vi "GFITS_WriteAmps.vi"(0 "fd":u64, 1 "filemsg":string, 2 "multimple extensions":bool, 3 "amplifiers":u64, 4 "eleRead":u32, 5 "error in":errorcluster, 6 "expID":string, 7 "Database RefNum in":T1, 8 "nodeID":string, 9 "headers":bool=TRUE, 10 "logfile":path, 11 "number of keywords":i32[](array[numeric])) -> (14 "file reference out":u64, 15 "return value":i32, 16 "after expID":string, 17 "image name out":string, 19 "error out":errorcluster)   [LabVIEW 2016]
uses:
  DBSHAND/private/vis/DatabaseHand_RefNum.ctl
  Common/public/vis/CMN_FVAR_action.ctl
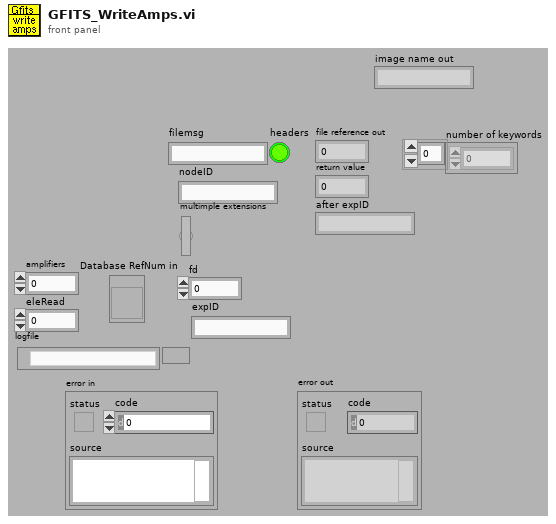
[diagram p1: front panel]
types:
  T1 = typedef "DatabaseHand_RefNum.ctl" = refnum<vi>
  T2 = typedef "CMN_FVAR_action.ctl" = enum16{"read", "write"}
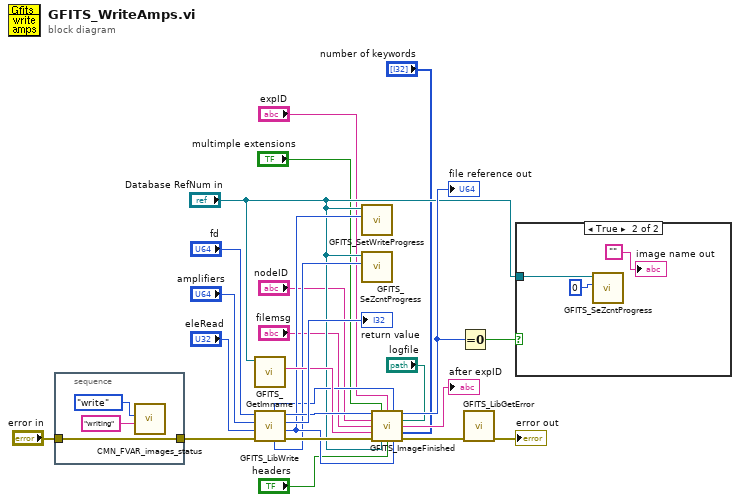
[diagram p0: block diagram]
diagram:
  n1 = stacked-sequence {
    tunnel: "error in" -> [w26]
    tunnel: [w26] -> w13
    frame #0 {
      n2 = call "CMN_FVAR_images_status.vi"("value in"="writing", "action"=CMN_FVAR_action."write") -> ()  [unwired: 9 out]
    }
  }
  n3 = call "GFITS_GetImname.vi"("Database RefNum"="Database RefNum in") -> ("name"=w21:string)  [unwired: 10 out]
  n4 = call "GFITS_LibWrite.vi"("error in (no error)"=w13, "eleRead"="eleRead", "amplifiers"="amplifiers", "fd"="fd") -> ("error out"=w24:errorcluster, "progress out"=w20:i32, "return value"=→"return value":i32, "fd out"=w23:u64, "zcnt out"=w17:i32, "num_amps"=w15:i32)  [unwired: 2 out]
  n5 = call "GFITS_SetWriteProgress.vi"("progress"=w20, "Database RefNum"="Database RefNum in") -> ()  [unwired: 1 in, 9 out]
  n6 = call "GFITS_SeZcntProgress.vi"("counter"=w17, "Database RefNum"="Database RefNum in") -> ()  [unwired: 1 in, 9 out]
  n7 = call "GFITS_ImageFinished.vi"("file reference"=w23, "multimple extensions"="multimple extensions", "_before_ expID"="expID", "num of extensions"=w15, "nodeID"="nodeID", "logfile"="logfile", "filemsg"="filemsg", "image name"=w21, "number of keywords"="number of keywords", "error in (no error)"=w24, "Database RefNum in"="Database RefNum in", "headers"="headers", "progress"=w20) -> ("file reference out"=w19:u64, "expID"=→"after expID":string, "error out"=w22:errorcluster)
  "file reference out" <- w19
  n8 = Equal To 0?(x=w19) -> (x = 0?=w18:bool)
  n9 = call "GFITS_LibGetError.vi"("error in (no error)"=w22) -> ("error out"=→"error out":errorcluster)  [unwired: 10 out]
  n10 = case shown="True" w18 {
    tunnel: "Database RefNum in" -> [_ w29]
    frame False {
    }
    frame True {
      n11 = call "GFITS_SeZcntProgress.vi"("counter"=0 ("zcount"), "Database RefNum"=w29) -> ()  [unwired: 1 in, 9 out]
      "image name out" <- ""
    }
  }
